vi "Core-Quit.vi"(8 "error in (no error)":errorcluster, 11 "Engine in":refnum<class "Engine.lvclass">) -> (0 "error out":errorcluster, 3 "Engine out":refnum<class "Engine.lvclass">)   [LabVIEW 2024, in "GLF.lvlib" / "Engine.lvclass"]
uses:
  Engine.lvclass
  Engine.lvclass/Engine.ctl
  <vilib>/Saukko/LV SDL3/Sources/SDL3/Init/Init.lvlib
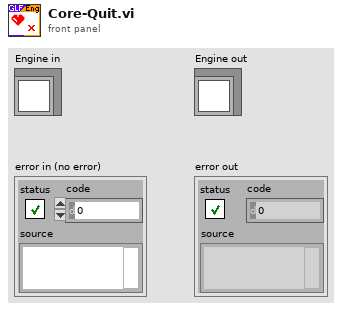
[diagram p1: front panel]
types:
  T1 = typedef "GLF.lvlib/Engine.lvclass/DVR--cluster.ctl" = cluster{"CMD Queue":T2, "Config":T3, "Ctxt":T5, "Metrics":T6}
  T2 = typedef "GLF.lvlib/Engine.lvclass/Command--queue.ctl" = refnum<queue>
  T3 = typedef "GLF.lvlib/Engine.lvclass/Config--cluster.ctl" = cluster{"Quit On Last Window Closed":bool, "VSync":T4, "FPS Target":dbl}
  T4 = typedef "GLF.lvlib/Engine.lvclass/VSync--enum.ctl" = enum16{"Disabled", "Enabled", "Adaptative"}
  T5 = typedef "GLF.lvlib/Engine.lvclass/Context--cluster.ctl" = cluster{"Ticks Begin":u64, "VSync Enabled":bool}
  T6 = typedef "GLF.lvlib/Engine.lvclass/Metrics--cluster.ctl" = cluster{"Uptime [ms]":u64, "Loop Time [ms]":u64}
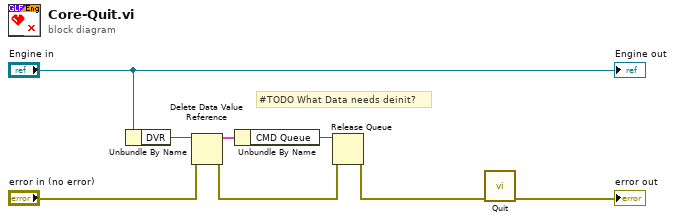
[diagram p0: block diagram]
diagram:
  # "#TODO What Data needs deinit?"
  n1 = Unbundle By Name("Engine in") -> ("DVR"=w5:refnum<data-value>)
  n2 = Delete Data Value Reference(data value reference=w5, error in="error in (no error)") -> (data value=w4:T1, error out=w1:errorcluster)
  n3 = Unbundle By Name(w4) -> ("CMD Queue"=w3:T2)
  n4 = Release Queue(queue=w3, error in (no error)=w1) -> (error out=w6:errorcluster)  [unwired: 1 in, 2 out]
  n5 = call <vilib>:"Quit.vi"("No Error"=w6) -> ("error out"=→"error out":errorcluster)  [unwired: 10 in]
  "Engine out" <- "Engine in"
